vi "Enable Controls.vi"(8 "error in (no error)":errorcluster, 10 "Disabled":T1(ring), 11 "Server in":refnum<class "Server.lvclass">) -> (0 "error out":errorcluster, 3 "Server out":refnum<class "Server.lvclass">)   [LabVIEW 2018, in "Server.lvlib" / "Server.lvclass"]
uses:
  Server.lvclass
  Server.lvclass/Server.ctl
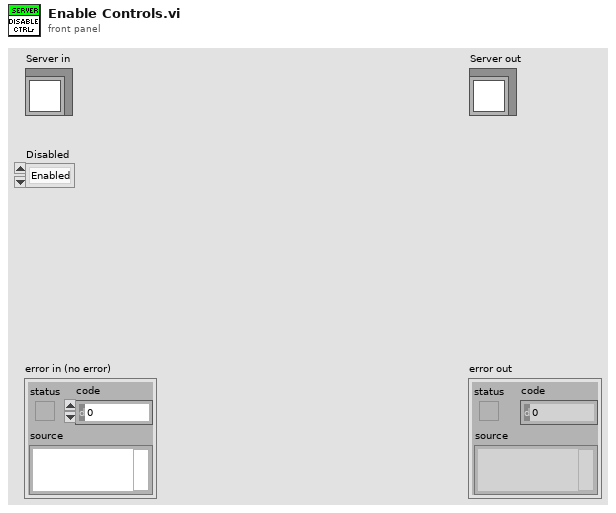
[diagram p1: front panel]
types:
  T1 = enum8{"Enabled", "Disabled", "Disabled and Grayed Out"}
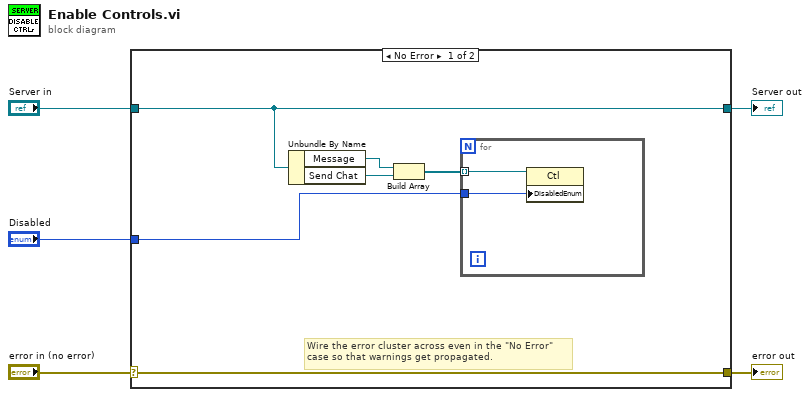
[diagram p0: block diagram]
diagram:
  n1 = case shown="No Error" "error in (no error)" {
    selector: "error in (no error)" -> [w11 w15]
    tunnel: [w11 w15] -> w4
    tunnel: [w10 w14] -> w2
    tunnel: "Server in" -> [w10 w14]
    tunnel: "Disabled" -> [w6 _]
    frame No Error {
      # "Wire the error cluster across even in the \"No Error\"\ncase so that warnings get propagated."
      n2 = Unbundle By Name(w10) -> ("Message"=w9:refnum<vi>, "Send Chat"=w8:refnum<vi>)
      n3 = Build Array(w9, w8) -> (w7:refnum<vi>[])
      n4 = for {
        tunnel: w7 -> [w13] mode=indexing
        tunnel: w6 -> [w12]
        n5 = property class="Ctl"(reference=w13, "DisabledEnum"=w12) -> ()  [unwired: 1 in, 2 out]
      }
    }
    frame Error {
    }
  }
  "error out" <- w4
  "Server out" <- w2
